vi "niRFUtil WFM Complex Differential (complex wfm).vi"(7 "Waveform In":T1 {"y" format="%.2f"; "dx" format="%^.2e"; "x0" format="%^.2e"}) -> (8 "Waveform Out":T1 {"y" format="%.2f"; "dx" format="%^.2e"; "x0" format="%^.2e"})   [LabVIEW 2015, in "niRFUtil.lvlib"]
doc: "(c) Copyright 2006, National Instruments, Inc. This VI may not be duplicated, sold, or distributed without written consent from National Instruments."
uses:
  niRFUtil.lvlib
  Includes/niRFUtil INC Complex Waveform.ctl
  Includes/niRFUtil INC Complex Array.ctl
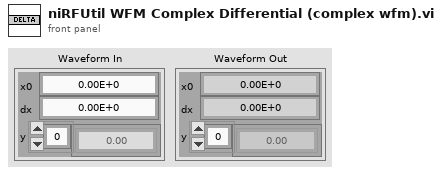
[diagram p1: front panel]
types:
  T1 = typedef "niRFUtil.lvlib/niRFUtil INC Complex Waveform.ctl" = cluster{"x0":dbl, "dx":dbl, "y":T2}
  T2 = typedef "niRFUtil.lvlib/niRFUtil INC Complex Array.ctl" = csg[]
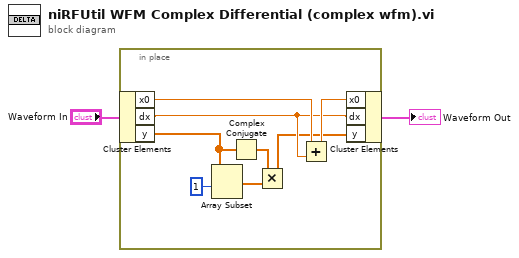
[diagram p0: block diagram]
diagram:
  n1 = in-place {
    n2 = in-place-cluster #1("Waveform In") -> ("x0"=w7:dbl, "dx"=w4:dbl, "y"=w6:T2)
    n3 = Array Subset(array=w6, index=1) -> (w9:T2)  [unwired: 1 in]
    n4 = Complex Conjugate(1:w6) -> (0:w8:T2)
    n5 = Multiply(x=w8, y=w9) -> (x*y=w3:T2)
    n6 = Add(x=w7, y=w4) -> (x+y=w5:dbl)
    n7 = in-place-cluster #1("x0"=w5, "dx"=w4, "y"=w3) -> (→"Waveform Out":T1)
  }
